vi "Timer Loop.vi"(8 "error in (no error)":errorcluster, 11 "Message Queues":T1) -> (0 "error out":errorcluster)   [LabVIEW 2014]
doc: "The message loop subVI to handle messages pertaining to logging data."
uses:
  support/Message Queue/All Message Queues.ctl
  Logging/Logging Configuration.ctl
  support/Message Queue/Enqueue Message (Single).vi
  <vilib>/Utility/error.llb/Error Cluster From Error Code.vi
  <vilib>/ErrorRing/Error Ring.xnode
  Logging/Logging.lvlib
  support/Message Queue/Message Queue.lvlib
  support/Message Queue/Message Cluster.ctl
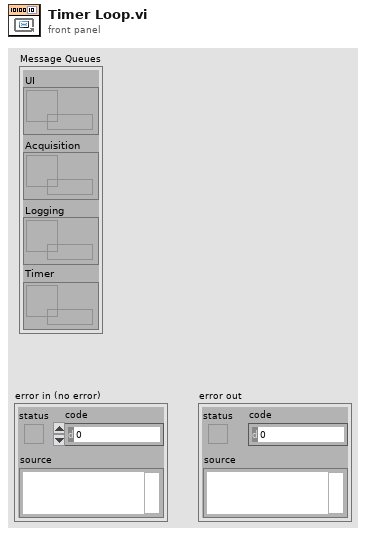
[diagram p1: front panel]
types:
  T1 = typedef "Message Queue.lvlib/All Message Queues.ctl" = cluster{"UI":refnum<queue>, "Acquisition":refnum<queue>, "Logging":refnum<queue>, "Timer":refnum<queue>}
  T2 = typedef "Logging.lvlib/Logging Configuration.ctl" = cluster{"Log File Base Path":path, "TDMS File Reference":refnum<k34>, "Samples to Save":u32, "InterRecording Delay":dbl}
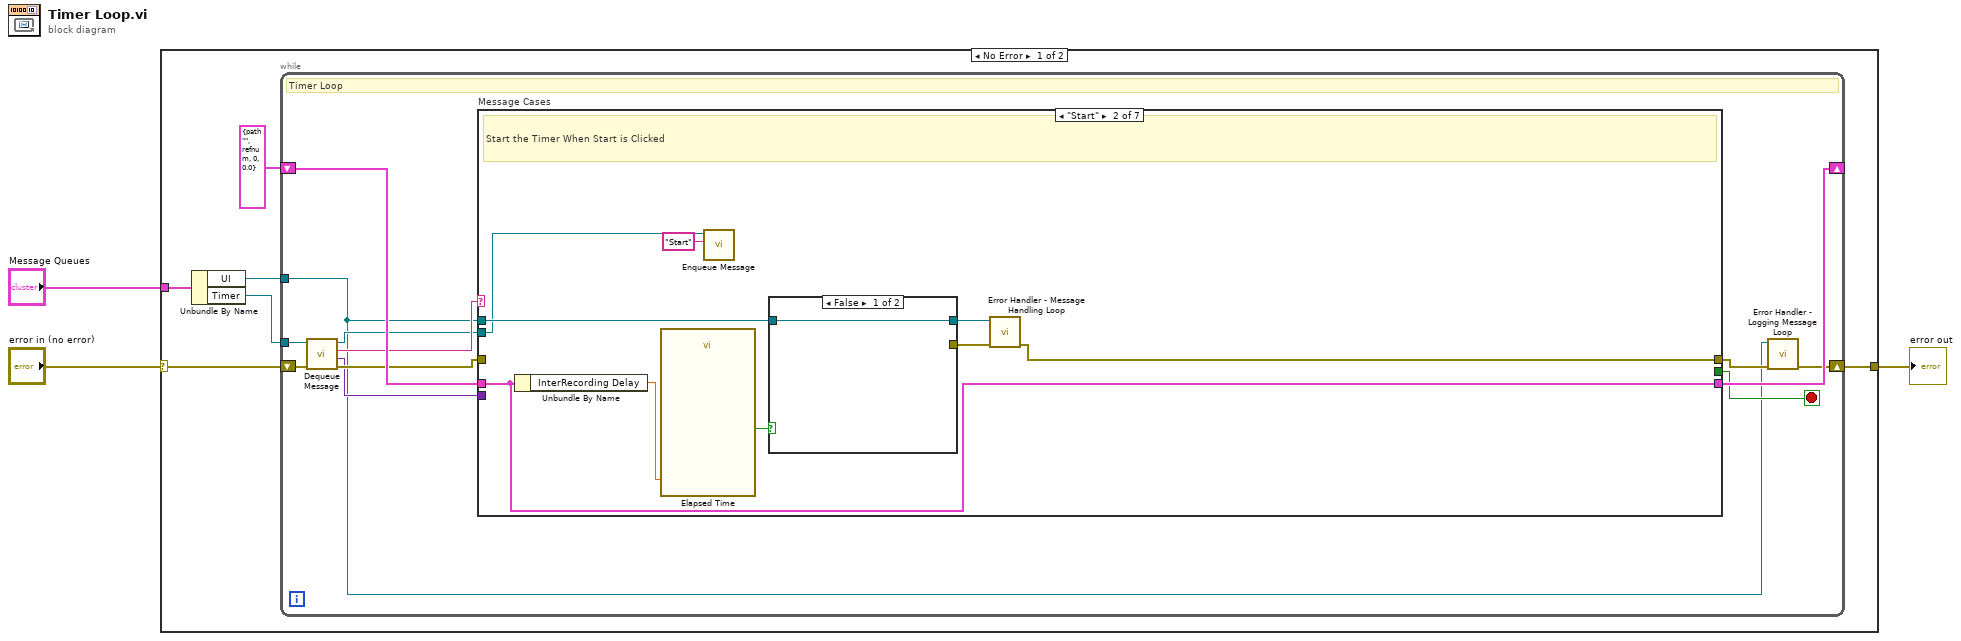
[diagram p0: block diagram]
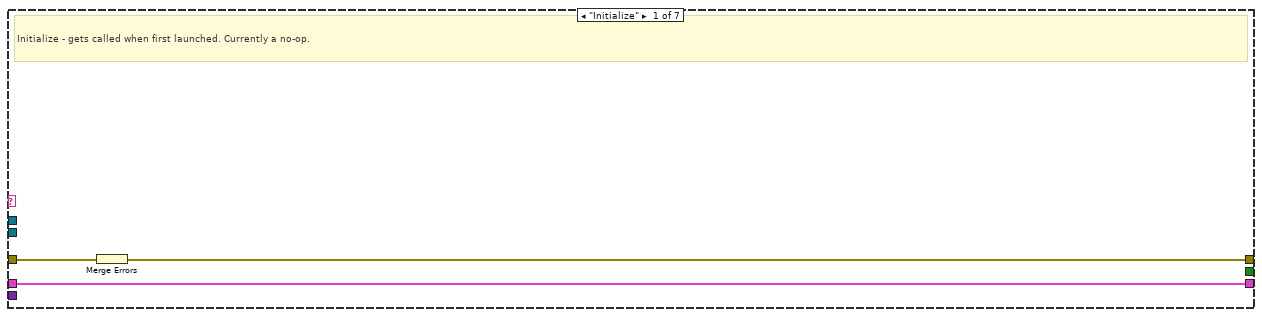
[diagram p2: hidden frame]
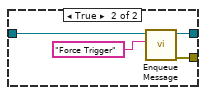
[diagram p3: hidden frame]
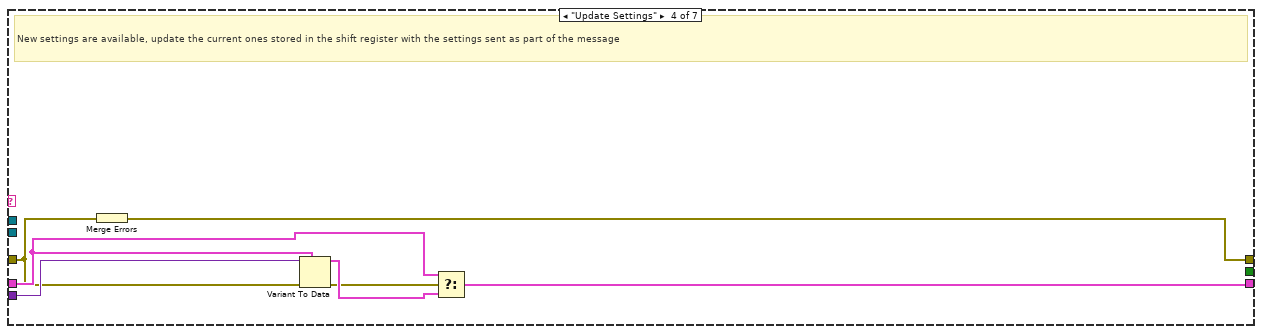
[diagram p5: hidden frame]
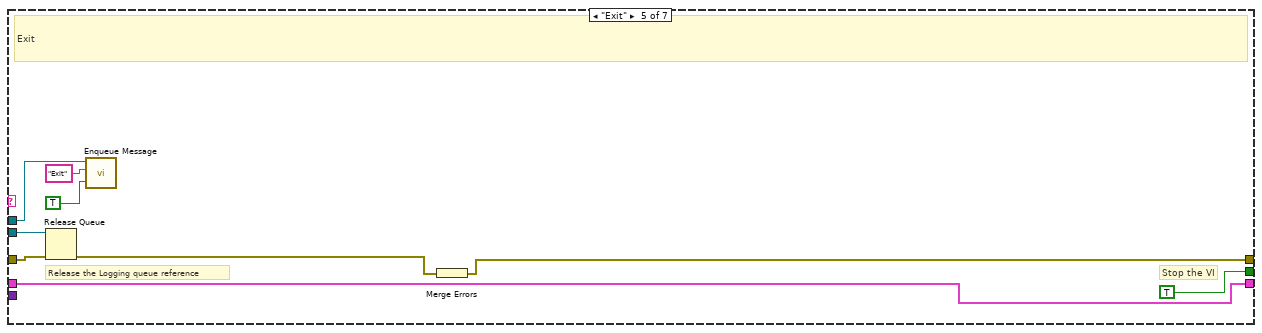
[diagram p6: hidden frame]
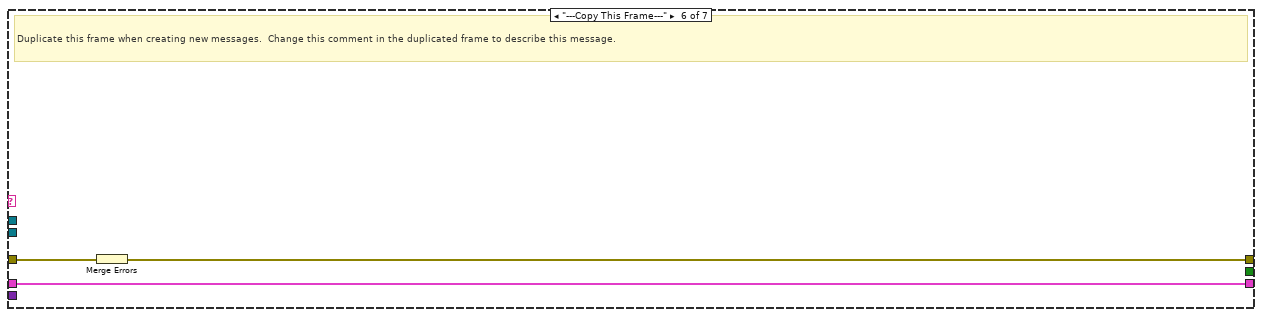
[diagram p7: hidden frame]
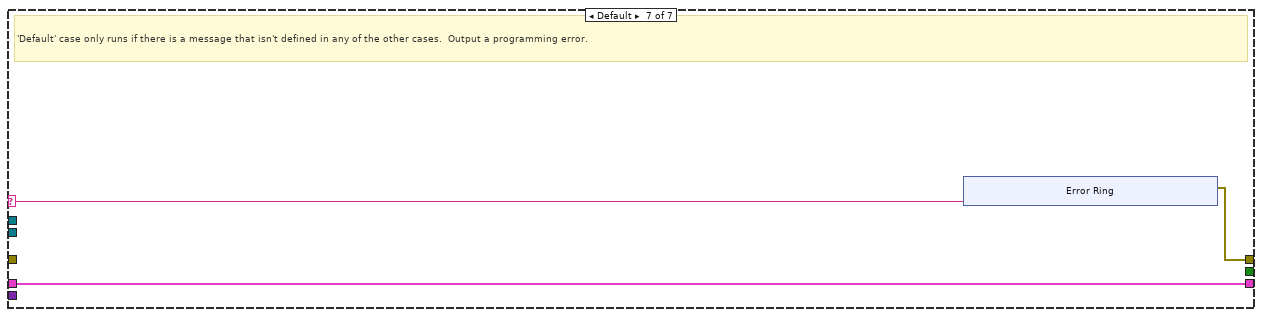
[diagram p8: hidden frame]
diagram:
  n1 = case shown="No Error" "error in (no error)" {
    selector: "error in (no error)" -> [w5 w70]
    tunnel: "Message Queues" -> [w9 _]
    tunnel: [w7 w70] -> w2
    frame No Error {
      n2 = Unbundle By Name(w9) -> ("UI"=w4:refnum<queue>, "Timer"=w8:refnum<queue>)
      n3 = while {
        tunnel: w8 -> [w13]
        shift-right: [w20] -> _
        shift-left: T2 {"Log File Base Path"=path "", "TDMS File Reference"=refnum, "Samples to Save"=0, "InterRecording Delay"=0.0} ("Logging Configuration") -> [w21]
        shift-right: [w11] -> w7
        shift-left: w5 -> [w18]
        tunnel: w4 -> [w10]
        stop <- w19 stop-if-true
        # "Timer Loop"
        n4 = call "Dequeue Message.vi"("error in (no error)"=w18, "Message Queue"=w13) -> ("error out"=w17:errorcluster, "Message Data"=w15:variant, "Message"=w16:string, "dup Message Queue"=w14:refnum<queue>)  [unwired: 6 in]
        n5 = case "Message Cases" shown="\"Start\"" w16 {
          selector: w16 -> [_ _ _ _ _ _ w60]
          tunnel: w14 -> [_ w26 _ _ w50 _ _]
          tunnel: w17 -> [w22 _ w39 w41 w53 w59 _]
          tunnel: [w24 w28 w39 w47 w55 w57 w61] -> w12
          tunnel: w21 -> [w23 w27 w40 w45 w49 w58 w62]
          tunnel: [w23 w27 w40 w42 w49 w58 w62] -> w20
          tunnel: [_ _ _ _ TRUE _ _] -> w19
          tunnel: w15 -> [_ _ _ w46 _ _ _]
          tunnel: w10 -> [_ w30 _ _ w54 _ _]
          frame "Initialize" {
            # "Initialize - gets called when first launched. Currently a no-op."
            n6 = Merge Errors(w22) -> (w24:errorcluster)
          }
          frame "Start" {
            # "Start the Timer When Start is Clicked"
            n7 = Unbundle By Name(w27) -> ("InterRecording Delay"=w29:dbl)
            n8 = call "Elapsed Time"("Time Target (s)"=w29) -> ("Time has Elapsed"=w33:bool)  [unwired: 11 in, 7 out]
            n9 = call-poly "Enqueue Message.vi"("Message"="Start", "Message Queue"=w26) -> ()  [unwired: 8 in, 2 out]
            n10 = case shown="False" w33 {
              tunnel: w30 -> [w34 w37]
              tunnel: [w34 w36] -> w32
              tunnel: [_ w35] -> w31
              frame False {
              }
              frame True {
                n11 = call-poly "Enqueue Message.vi"("Message"="Force Trigger", "Message Queue"=w37) -> ("error out"=w35:errorcluster, "dup Message Queue"=w36:refnum<queue>)  [unwired: 8 in]
              }
            }
            n12 = call "Error Handler - Message Handling Loop.vi"("error in (no error)"=w31, "Message Queue"=w32) -> ("dup error in"=w28:errorcluster)  [unwired: 8 in, 1 out]
          }
          frame "Stop" {
            # "Stop - Flush the message queue of any pending \"Log\" messages. Call 'Flush Data to Log File.vi' so any pending data is not lost."
          }
          frame "Update Settings" {
            # "New settings are available, update the current ones stored in the shift register with the settings sent as part of the message"
            n13 = Merge Errors(w41) -> (w47:errorcluster)
            n14 = Variant To Data(error in=w41, type=w45, Variant=w46) -> (data=w44:T2, error out=w43:errorcluster)
            n15 = Select(t=w45, s=w43, f=w44) -> (s? t:f=w42:T2)
          }
          frame "Exit" {
            # "Release the Logging queue reference"
            # "Stop the VI"
            # "Exit"
            n16 = Release Queue(queue=w50, error in (no error)=w53) -> (error out=w48:errorcluster)  [unwired: 1 in, 2 out]
            n17 = call-poly "Enqueue Message.vi"("Priority Message? (F)"=TRUE, "Message"="Exit", "Message Queue"=w54) -> ()  [unwired: 7 in, 2 out]
            n18 = Merge Errors(w48) -> (w55:errorcluster)
          }
          frame "---Copy This Frame---" {
            # "Duplicate this frame when creating new messages.  Change this comment in the duplicated frame to describe this message."
            n19 = Merge Errors(w59) -> (w57:errorcluster)
          }
          frame Default {
            # "'Default' case only runs if there is a message that isn't defined in any of the other cases.  Output a programming error."
            n20 = xnode "Error Ring"("parameter 0"=w60) -> ("error out"=w61:errorcluster)
          }
        }
        n21 = call "Error Handler - Logging Message Loop.vi"("error in (no error)"=w12, "Message Queue"=w10) -> ("dup error in"=w11:errorcluster)  [unwired: 8 in, 1 out]
      }
    }
    frame Error {
    }
  }
  "error out" <- w2
